vi "Close.vi"(8 "error in":errorcluster, 10 "configuration":T1, 11 "session":T2) -> (0 "error out":errorcluster)   [LabVIEW 2021, in "dcvmDPI_AD7606B_serverImpl.lvlib"]
uses:
  dcvmDPI_AD7606B_serverImpl.lvlib
  controls/session.ctl
  controls/configuration.ctl
  <vilib>/FPGAPlugInAG/Dynamic/niLvFpga_Close_Dynamic.vi
  <vilib>/rvi/interface/nirviCloseFPGA/nirviCloseFPGA.xnode
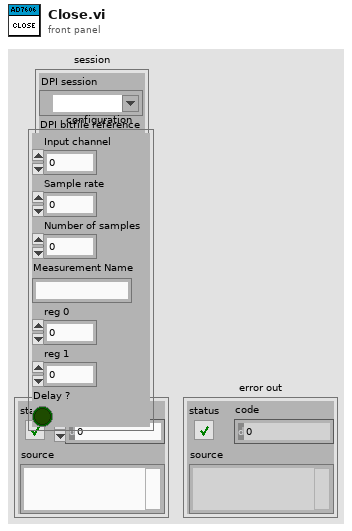
[diagram p1: front panel]
types:
  T1 = typedef "dcvmDPI_AD7606B_serverImpl.lvlib/configuration.ctl" = cluster{"Input channel":i32, "Sample rate":dbl, "Number of samples":u32, "Measurement Name":string, "reg 0":i32, "reg 1":i32, "Delay ?":bool}
  T2 = typedef "dcvmDPI_AD7606B_serverImpl.lvlib/session.ctl" = cluster{"DPI session":refnum<k15>, "DPI bitfile reference":refnum<k20>}
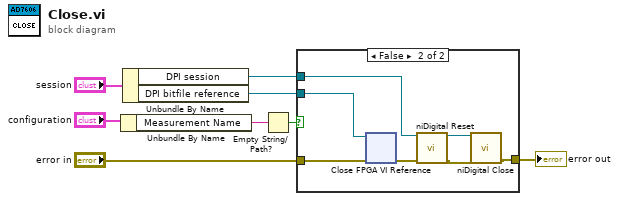
[diagram p0: block diagram]
diagram:
  n1 = Unbundle By Name("configuration") -> ("Measurement Name"=w7:string)
  n2 = Unbundle By Name("session") -> ("DPI session"=w5:refnum<k15>, "DPI bitfile reference"=w4:refnum<k20>)
  n3 = Empty String/Path?(string/path=w7) -> (empty?=w1:bool)
  n4 = case shown="False" w1 {
    tunnel: w5 -> [_ w12]
    tunnel: w4 -> [_ w13]
    tunnel: "error in" -> [w9 w11]
    tunnel: [w9 w10] -> w2
    frame True {
    }
    frame False {
      n5 = xnode "Close FPGA VI Reference"("FPGA VI Reference In"=w13, "error in"=w11) -> ("error out"=w14:errorcluster)
      n6 = call <instrlib>:"niDigital Reset.vi"("instrument handle in"=w12, "error in"=w14) -> ("instrument handle out"=w16:refnum<k15>, "error out"=w15:errorcluster)  [unwired: 12 in]
      n7 = call <instrlib>:"niDigital Close.vi"("instrument handle"=w16, "error in"=w15) -> ("error out"=w10:errorcluster)  [unwired: 13 in]
    }
  }
  "error out" <- w2
